vi "FGV Test Timer.vi"(11 "FGV Test Time":T1) -> (3 "Time (s)":dbl)   [LabVIEW 2021]
uses:
  FGV Test Time Action.ctl
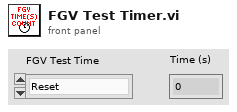
[diagram p1: front panel]
types:
  T1 = typedef "FGV Test Time Action.ctl" = enum16{"Reset", "Read"}
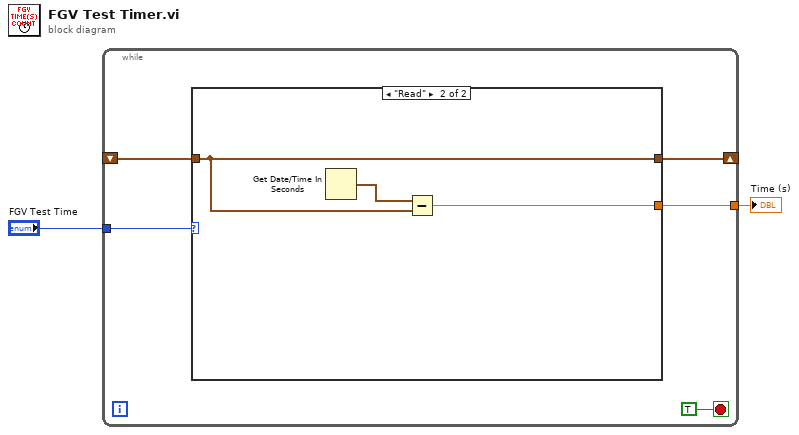
[diagram p0: block diagram]
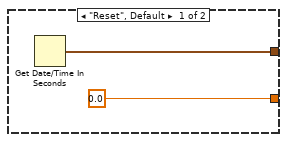
[diagram p2: hidden frame]
diagram:
  n1 = while {
    tunnel: "FGV Test Time" -> [w6]
    tunnel: [w5] -> w1
    shift-right: [w4] -> _
    shift-left: _ -> [w3]
    stop <- TRUE stop-if-true
    n2 = case shown="\"Read\"" w6 {
      tunnel: [0.0 w11] -> w5
      tunnel: [w8 w10] -> w4
      tunnel: w3 -> [_ w10]
      frame "Reset", Default {
        n3 = Get Date/Time In Seconds() -> (seconds since 1Jan1904=w8:timestamp)
      }
      frame "Read" {
        n4 = Get Date/Time In Seconds() -> (seconds since 1Jan1904=w12:timestamp)
        n5 = Subtract(x=w12, y=w10) -> (x-y=w11:dbl)
      }
    }
  }
  "Time (s)" <- w1
